vi "python_and_motors.vi"() -> ()   [LabVIEW 2019]
uses:
  <vilib>/addons/eal4LabVIEW/ApiLib/Connection control/ealApiConnect_string.vi
  <vilib>/addons/eal4LabVIEW/eal4LabVIEW.lvlib
panel:
  in  "stop":bool
  out "rpm motor 1":dbl
  in  "condition 1":i32(ring) items=["AXIS_CONDITION_ACTIVE"=0, "AXIS_CONDITION_PARKING"=1, "AXIS_CONDITION_DEACTIVATED"=2, "AXIS_CONDITION_ACTIVE_DECOUPLED"=4, "AXIS_CONDITION_PARKING_DECOUPLED"=5, "AXIS_CONDITION_DEACTIVATED_DECOUPLED"=6, "AXIS_CONDITION_ACTIVE_PARAMETERIZATION"=8, "AXIS_CONDITION_PARKING_PARAMETERIZATION"=9, "AXIS_CONDITION_DEACTIVATED_PARAMETERIZATION"=10, "AXIS_CONDITION_ACTIVE_DECOUPLED_PARAMETERIZATION"=12, "AXIS_CONDITION_PARKING_DECOUPLED_PARAMETERIZATION"=13, "AXIS_CONDITION_DEACTIVATED_DECOUPLED_PARAMETERIZATION"=14]
  in  "slave index 1":i32
  in  "condition 2":i32(ring) items=["AXIS_CONDITION_ACTIVE"=0, "AXIS_CONDITION_PARKING"=1, "AXIS_CONDITION_DEACTIVATED"=2, "AXIS_CONDITION_ACTIVE_DECOUPLED"=4, "AXIS_CONDITION_PARKING_DECOUPLED"=5, "AXIS_CONDITION_DEACTIVATED_DECOUPLED"=6, "AXIS_CONDITION_ACTIVE_PARAMETERIZATION"=8, "AXIS_CONDITION_PARKING_PARAMETERIZATION"=9, "AXIS_CONDITION_DEACTIVATED_PARAMETERIZATION"=10, "AXIS_CONDITION_ACTIVE_DECOUPLED_PARAMETERIZATION"=12, "AXIS_CONDITION_PARKING_DECOUPLED_PARAMETERIZATION"=13, "AXIS_CONDITION_DEACTIVATED_DECOUPLED_PARAMETERIZATION"=14]
  in  "slave index 2":i32
  out "rpm motor 2":dbl
  out "rpm motor 3":dbl
  in  "condition 3":i32(ring) items=["AXIS_CONDITION_ACTIVE"=0, "AXIS_CONDITION_PARKING"=1, "AXIS_CONDITION_DEACTIVATED"=2, "AXIS_CONDITION_ACTIVE_DECOUPLED"=4, "AXIS_CONDITION_PARKING_DECOUPLED"=5, "AXIS_CONDITION_DEACTIVATED_DECOUPLED"=6, "AXIS_CONDITION_ACTIVE_PARAMETERIZATION"=8, "AXIS_CONDITION_PARKING_PARAMETERIZATION"=9, "AXIS_CONDITION_DEACTIVATED_PARAMETERIZATION"=10, "AXIS_CONDITION_ACTIVE_DECOUPLED_PARAMETERIZATION"=12, "AXIS_CONDITION_PARKING_DECOUPLED_PARAMETERIZATION"=13, "AXIS_CONDITION_DEACTIVATED_DECOUPLED_PARAMETERIZATION"=14]
  in  "slave index 3":i32
  out "return value":dbl[](array[numeric])
  out "Iteration counter":i32
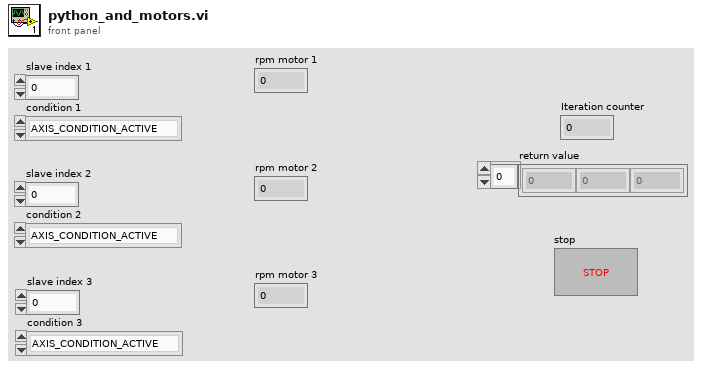
[diagram p1: front panel]
types:
  T1 = cluster{"Velocity":dbl, "Acceleration":dbl, "Deceleration":dbl, "Jerk":dbl}
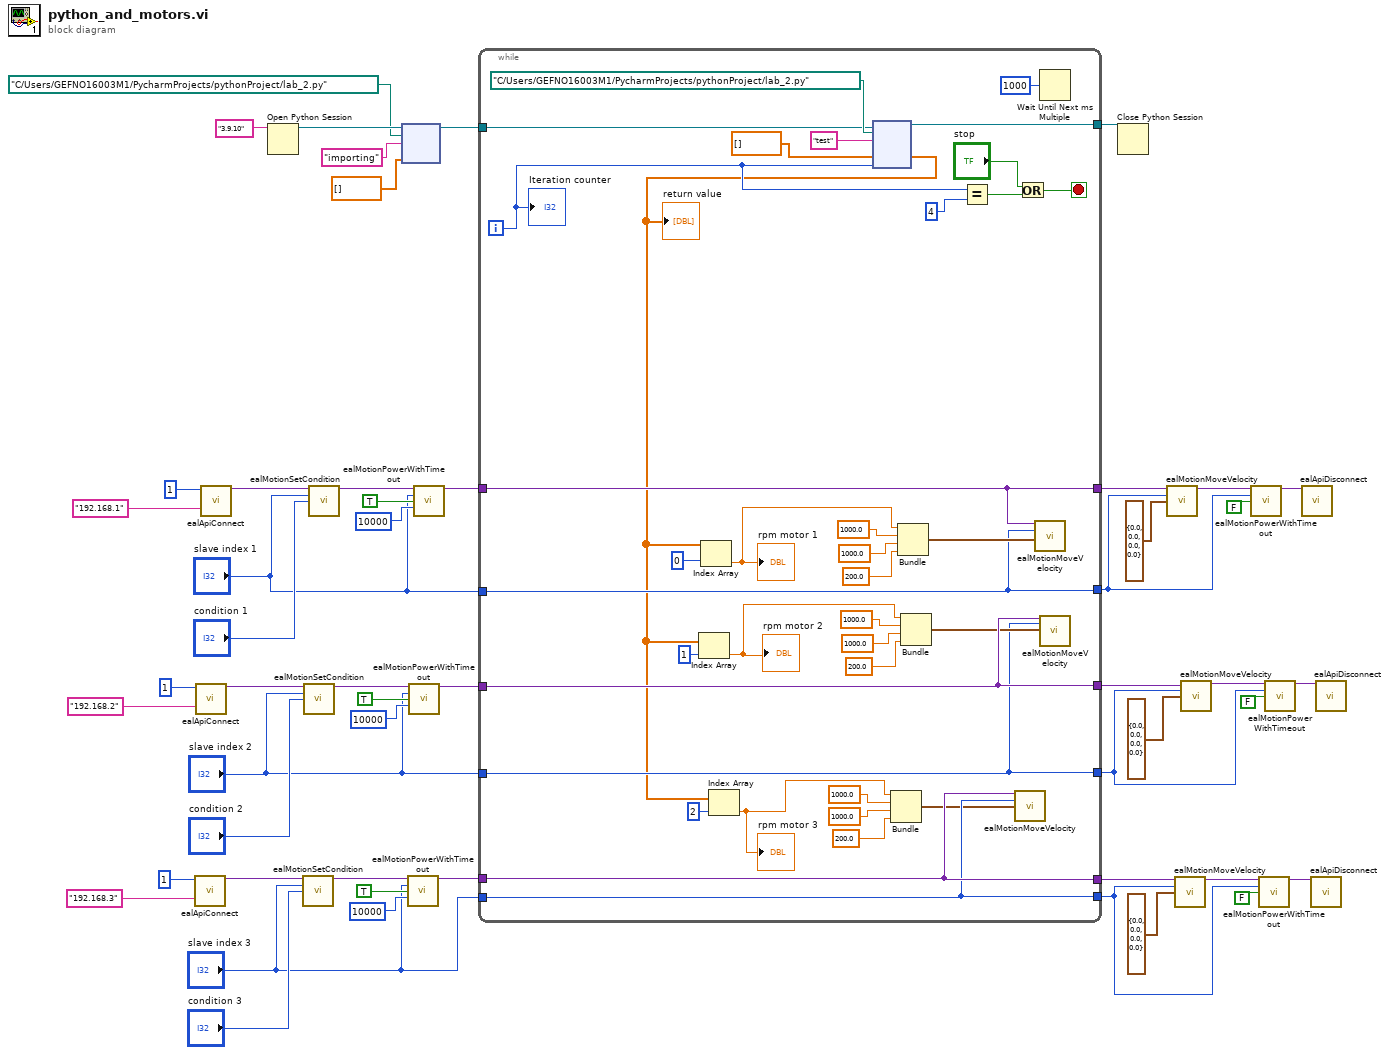
[diagram p0: block diagram]
diagram:
  n1 = call-poly <vilib>:"ealApiConnect.vi"("maximum no of axes"=1, "ip address"="192.168.3") -> ("connection out"=w43:variant)  [unwired: 12 in, 1 out]
  n2 = call-poly <vilib>:"ealApiConnect.vi"("maximum no of axes"=1, "ip address"="192.168.2") -> ("connection out"=w29:variant)  [unwired: 12 in, 1 out]
  n3 = call-poly <vilib>:"ealApiConnect.vi"("maximum no of axes"=1, "ip address"="192.168.1") -> ("connection out"=w15:variant)  [unwired: 12 in, 1 out]
  n4 = Open Python Session(python version="3.9.10" ("Python version")) -> (session out=w52:refnum<k35>)  [unwired: 2 in, 1 out]
  n5 = call <vilib>:"ealMotionSetCondition.vi"("connection in"=w43, "slave index"="slave index 3", "condition"="condition 3") -> ("connection out"=w42:variant)  [unwired: 11 in, 1 out]
  n6 = call <vilib>:"ealMotionSetCondition.vi"("connection in"=w29, "slave index"="slave index 2", "condition"="condition 2") -> ("connection out"=w28:variant)  [unwired: 11 in, 1 out]
  n7 = call <vilib>:"ealMotionSetCondition.vi"("connection in"=w15, "slave index"="slave index 1", "condition"="condition 1") -> ("connection out"=w14:variant)  [unwired: 11 in, 1 out]
  n8 = node(w52, path "C:/Users/GEFNO16003M1/PycharmProjects/pythonProject/lab_2.py" ("module path"), "importing" ("function name"), dbl[] []) -> (w46:refnum<k35>)  [unwired: 2 in, 3 out]
  n9 = call <vilib>:"ealMotionPowerWithTimeout.vi"("connection in"=w42, "slave index"="slave index 3", "value"=TRUE, "timeout"=10000) -> ("connection out"=w38:variant)  [unwired: 10 in, 1 out]
  n10 = call <vilib>:"ealMotionPowerWithTimeout.vi"("connection in"=w28, "slave index"="slave index 2", "value"=TRUE, "timeout"=10000) -> ("connection out"=w20:variant)  [unwired: 10 in, 1 out]
  n11 = call <vilib>:"ealMotionPowerWithTimeout.vi"("connection in"=w14, "slave index"="slave index 1", "value"=TRUE, "timeout"=10000) -> ("connection out"=w6:variant)  [unwired: 10 in, 1 out]
  n12 = while {
    tunnel: [w88] -> w48
    tunnel: w46 -> [w84]
    tunnel: w38 -> [w81]
    tunnel: [w81] -> w36
    tunnel: "slave index 3" -> [w80]
    tunnel: [w80] -> w32
    tunnel: w20 -> [w73]
    tunnel: [w73] -> w19
    tunnel: "slave index 2" -> [w66]
    tunnel: [w66] -> w18
    tunnel: w6 -> [w62]
    tunnel: [w62] -> w5
    tunnel: "slave index 1" -> [w58]
    tunnel: [w58] -> w1
    i -> [w57]
    stop <- w56 stop-if-true
    n13 = node(w84, path "C:/Users/GEFNO16003M1/PycharmProjects/pythonProject/lab_2.py" ("module path"), "test" ("function name"), dbl[] [], w57) -> (w88:refnum<k35>, w53:dbl[])  [unwired: 2 in, 3 out]
    "return value" <- w53
    n14 = Index Array(array=w53, index=1) -> (element=w67:dbl)
    "rpm motor 2" <- w67
    n15 = Index Array(array=w53, index=0) -> (element=w61:dbl)
    "rpm motor 1" <- w61
    n16 = Index Array(array=w53, index=2) -> (element=w74:dbl)
    "rpm motor 3" <- w74
    n17 = Bundle(w74, 1000.0, 1000.0, 200.0) -> (w75:cluster{dbl, dbl, dbl, dbl})  [unwired: 1 in]
    n18 = Bundle(w61, 1000.0, 1000.0, 200.0) -> (w59:cluster{dbl, dbl, dbl, dbl})  [unwired: 1 in]
    n19 = Bundle(w67, 1000.0, 1000.0, 200.0) -> (w68:cluster{dbl, dbl, dbl, dbl})  [unwired: 1 in]
    n20 = Equal?(x=w57, y=4) -> (x = y?=w54:bool)
    n21 = call <vilib>:"ealMotionMoveVelocity.vi"("connection in"=w81, "slave index"=w80, "parameters set"=w75) -> ()  [unwired: 11 in, 2 out]
    n22 = Or(x="stop", y=w54) -> (x .or. y?=w56:bool)
    n23 = call <vilib>:"ealMotionMoveVelocity.vi"("connection in"=w62, "slave index"=w58, "parameters set"=w59) -> ()  [unwired: 11 in, 2 out]
    n24 = Wait Until Next ms Multiple(millisecond multiple=u32 1000) -> ()  [unwired: 1 out]
    n25 = call <vilib>:"ealMotionMoveVelocity.vi"("connection in"=w73, "slave index"=w66, "parameters set"=w68) -> ()  [unwired: 11 in, 2 out]
    "Iteration counter" <- w57
  }
  n26 = Close Python Session(session in=w48) -> ()  [unwired: 1 in, 1 out]
  n27 = call <vilib>:"ealMotionMoveVelocity.vi"("connection in"=w5, "slave index"=w1, "parameters set"=T1 {"Velocity"=0.0, "Acceleration"=0.0, "Deceleration"=0.0, "Jerk"=0.0}) -> ("connection out"=w9:variant)  [unwired: 11 in, 1 out]
  n28 = call <vilib>:"ealMotionMoveVelocity.vi"("connection in"=w36, "slave index"=w32, "parameters set"=T1 {"Velocity"=0.0, "Acceleration"=0.0, "Deceleration"=0.0, "Jerk"=0.0}) -> ("connection out"=w35:variant)  [unwired: 11 in, 1 out]
  n29 = call <vilib>:"ealMotionMoveVelocity.vi"("connection in"=w19, "slave index"=w18, "parameters set"=T1 {"Velocity"=0.0, "Acceleration"=0.0, "Deceleration"=0.0, "Jerk"=0.0}) -> ("connection out"=w23:variant)  [unwired: 11 in, 1 out]
  n30 = call <vilib>:"ealMotionPowerWithTimeout.vi"("connection in"=w9, "slave index"=w1, "value"=FALSE) -> ("connection out"=w10:variant)  [unwired: 11 in, 1 out]
  n31 = call <vilib>:"ealMotionPowerWithTimeout.vi"("connection in"=w35, "slave index"=w32, "value"=FALSE) -> ("connection out"=w37:variant)  [unwired: 11 in, 1 out]
  n32 = call <vilib>:"ealMotionPowerWithTimeout.vi"("connection in"=w23, "slave index"=w18, "value"=FALSE) -> ("connection out"=w24:variant)  [unwired: 11 in, 1 out]
  n33 = call <vilib>:"ealApiDisconnect.vi"("connection in"=w10) -> ()  [unwired: 14 in, 1 out]
  n34 = call <vilib>:"ealApiDisconnect.vi"("connection in"=w37) -> ()  [unwired: 14 in, 1 out]
  n35 = call <vilib>:"ealApiDisconnect.vi"("connection in"=w24) -> ()  [unwired: 14 in, 1 out]
